vi "ReadContent.vi"(8 "error in (no error)":errorcluster, 11 "object in":refnum<class "Message Class.lvclass">) -> (0 "error out":errorcluster, 2 "content":variant, 3 "object out":refnum<class "Message Class.lvclass">)   [LabVIEW 2018, in "ClientMessaging.lvlib" / "Message Class.lvclass"]
uses:
  Message Class.lvclass
  Message Class.lvclass/Message Class.ctl
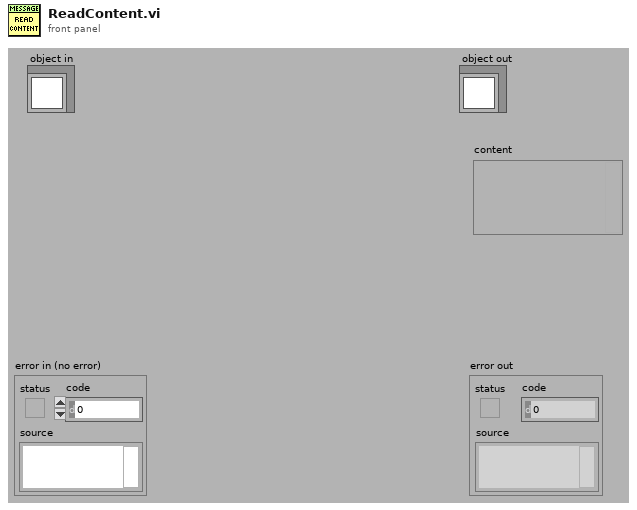
[diagram p1: front panel]
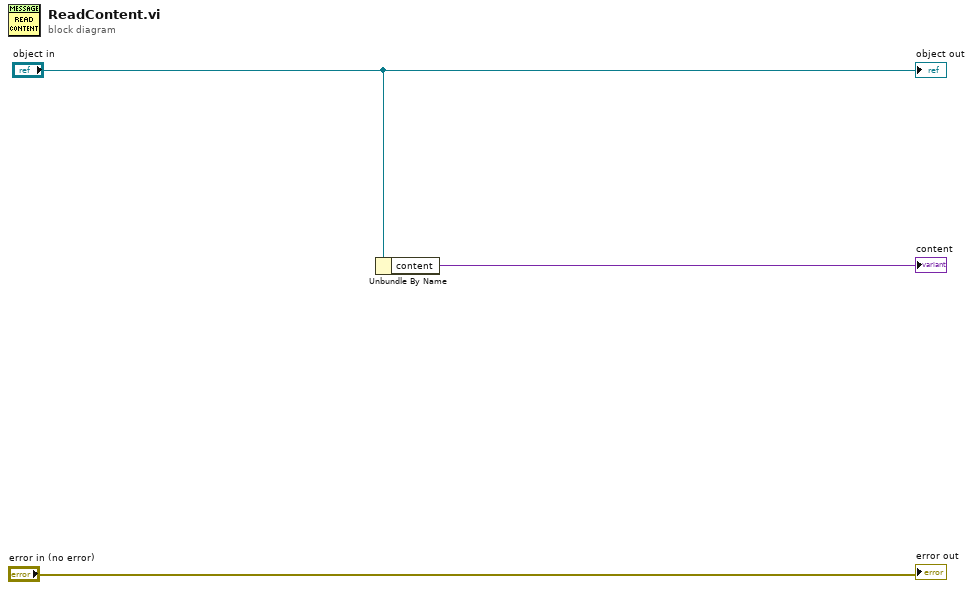
[diagram p0: block diagram]
diagram:
  n1 = Unbundle By Name("object in") -> ("content"=→"content":variant)
  "error out" <- "error in (no error)"
  "object out" <- "object in"
